vi "PSD.vi"(8 "error in (no error)":errorcluster, 9 "Save Spectrum":bool, 10 "Python version":string, 11 "data":waveform(dbl)[](array[waveform])) -> (0 "error out":errorcluster, 3 "Array":cluster{dbl, dbl, dbl[]}[](array[cluster]))   [LabVIEW 2019]
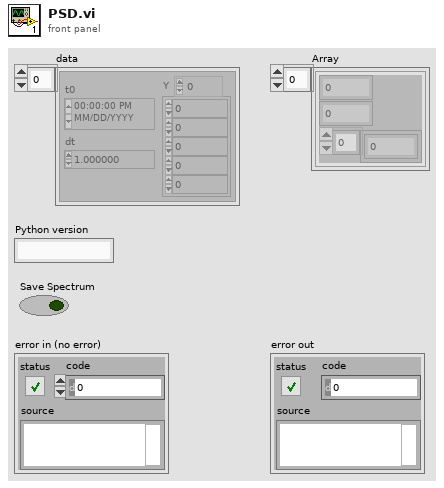
[diagram p1: front panel]
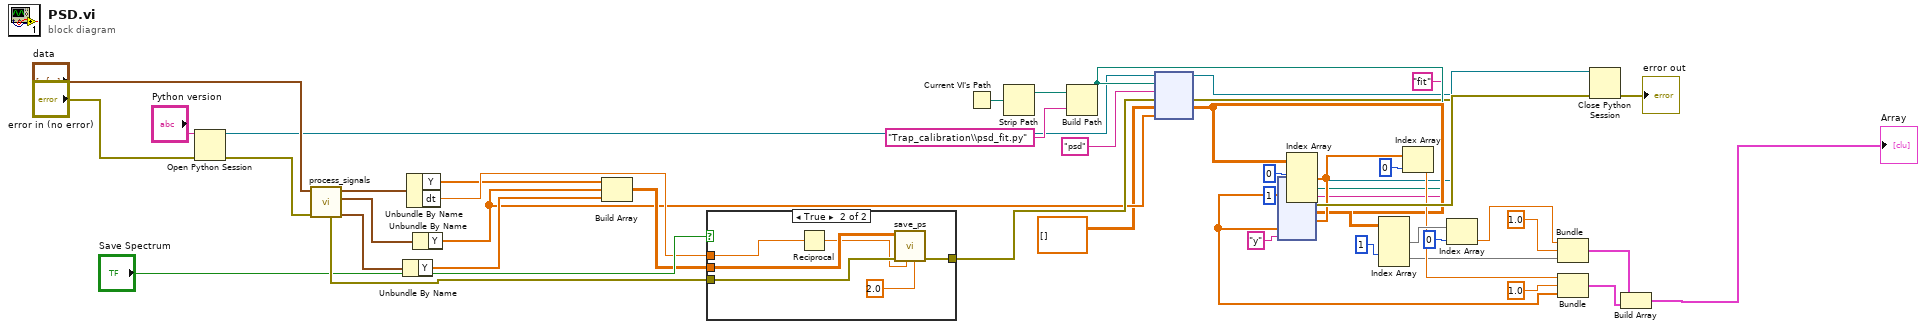
[diagram p0: block diagram]
diagram:
  n1 = Open Python Session(python version="Python version", 3:"error in (no error)") -> (session out=w2:refnum<k35>, error out=w45:errorcluster)  [unwired: 1 in]
  n2 = call "process_signals.vi"("error in (no error)"=w45, "data"="data") -> ("SUM"=w33:waveform(dbl), "BT"=w6:waveform(dbl), "LR"=w32:waveform(dbl), "error out"=w40:errorcluster)  [unwired: 5 in, 1 out]
  n3 = Unbundle By Name(w33) -> ("Y"=w36:dbl[])
  n4 = Unbundle By Name(w32) -> ("Y"=w34:dbl[], "dt"=w38:dbl)
  n5 = Unbundle By Name(w6) -> ("Y"=w35:dbl[])
  n6 = Build Array(w34, w35, w36) -> (w37:dbl[][])
  n7 = case shown="True" "Save Spectrum" {
    tunnel: w37 -> [_ w53]
    tunnel: w38 -> [_ w50]
    tunnel: w40 -> [w48 w52]
    tunnel: [w48 w51] -> w41
    frame False {
    }
    frame True {
      n8 = Reciprocal(x=w50) -> (1/x=w49:dbl)
      n9 = call "save_ps.vi"("Height"=2.0, "Rate"=w49, "error in"=w52, "QPD Data"=w53) -> ("error out"=w51:errorcluster)  [unwired: 7 in]
    }
  }
  n10 = Current VI's Path() -> (path=w8:path)
  n11 = Strip Path(path=w8) -> (stripped path=w9:path)  [unwired: 1 out]
  n12 = Build Path(base path=w9, name or relative path="Trap_calibration\\psd_fit.py") -> (appended path=w16:path)
  n13 = node(w2, w16, "psd" ("function name"), w41, dbl[][] [], w35) -> (w12:refnum<k35>, w14:errorcluster, w17:dbl[][])  [unwired: 1 in, 2 out]
  n14 = Index Array(array=w17, index (row) #1=0 ("index (row)"), index (row) #2=1 ("index (row)")) -> (element #1=w24:dbl[], element #2=w18:dbl[])  [unwired: 2 in]
  n15 = node(w12, w16, "fit" ("function name"), w14, w17, w24, w18, "y" ("function name")) -> (w13:refnum<k35>, w46:errorcluster, w21:dbl[][])  [unwired: 3 in, 2 out]
  n16 = Index Array(array=w21, index (row) #2=1 ("index (row)")) -> (element #1=w27:dbl[], element #2=w22:dbl[])  [unwired: 3 in]
  n17 = Index Array(array=w24, index=0) -> (element=w26:dbl)
  n18 = Index Array(array=w27, index=0) -> (element=w30:dbl)
  n19 = Bundle(w30, 1.0, w22) -> (w42:cluster{dbl, dbl, dbl[]})  [unwired: 1 in]
  n20 = Bundle(w26, 1.0, w18) -> (w43:cluster{dbl, dbl, dbl[]})  [unwired: 1 in]
  n21 = Close Python Session(session in=w13, error in=w46) -> (11:→"error out":errorcluster)
  n22 = Build Array(w42, w43) -> (→"Array":cluster{dbl, dbl, dbl[]}[])
